vi "Rubix Cube Main.vi"() -> (0 "Rbt cmd":string)   [LabVIEW 2019]
uses:
  left arrow.ctl
  down arrow.ctl
  right arrow.ctl
  up arrow.ctl
  rotate right.ctl
  rotate left.ctl
  TCP send commands.ctl
  UI Mode.ctl
  error module commands.ctl
  Stop Timing Module commands.vi
  main queue data type.ctl
  top level commands.ctl
  Cube Data Ops.ctl
  facet and command.ctl
  Play timing module commands.ctl
  Scene Commands.ctl
  Robot Movement Command Interpreter - to robot.vi
  preform rotate op -numeric.vi
  Robot Movement Command Interpreter - to rubix.vi
panel:
  out "Array":u16[][](array[numeric])=[[1, 5, 2, 4, 3, 5, 4, 2, 3], [0, 5, 4, 1, 2, 0, 5, 2, 2], [1, 2, 1, 1, 0, 0, 4, 1, 4], [3, 4, 0, 4, 1, 1, 2, 4, 3], [5, 3, 0, 2, 5, 3, 5, 0, 5], [1, 5, 2, 3, 4, 0, 0, 3, 3]]
  in  "Sync to Cube":bool
  in  "Rotation Resolution":dbl=10.0
  in  "Go To face":bool
  in  "Solve":bool
  in  "Test":bool
  in  "Difficulty":u16(ring)=5 items=["Easy"=5, "Medium"=20, "Hard"=50, "Challenge"=100]
  in  "Randomize":bool
  in  "Game Play Type":enum16{"Standalone", "UI Master", "UI Salve"}(ring)
  in  "Face":u8=1 min=1 max=6 step=1
  in  "Face ccw":T1
  in  "Face cw":T2
  in  "Right column up":T3
  in  "Middle column up":T3
  in  "Left column up":T3
  in  "Bottom row right":T4
  in  "Middle row right":T4
  in  "Top row right":T4
  in  "Right column down":T5
  in  "Middle column down":T5
  in  "Left column down":T5
  in  "Bottom row left":T6
  in  "Middle row left":T6
  in  "Top row left":T6
  in  "stop":bool
  # "Aux Functions (do not use)"
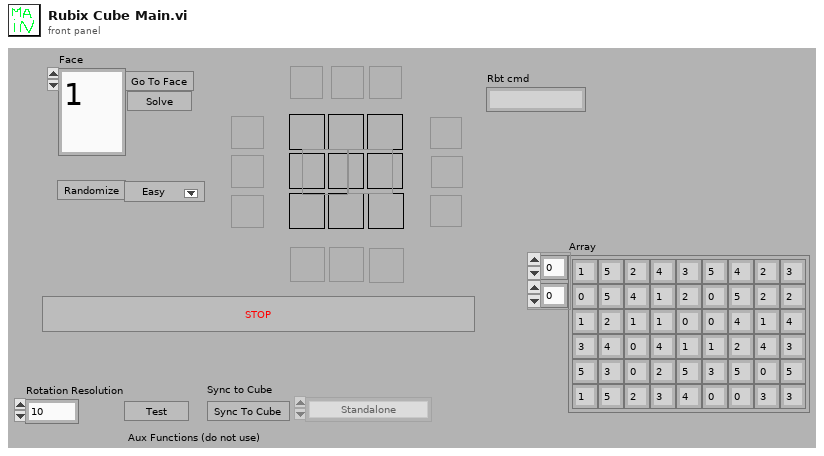
[diagram p1: front panel]
types:
  T1 = typedef "rotate left.ctl" = bool
  T2 = typedef "rotate right.ctl" = bool
  T3 = typedef "up arrow.ctl" = bool
  T4 = typedef "right arrow.ctl" = bool
  T5 = typedef "down arrow.ctl" = bool
  T6 = typedef "left arrow.ctl" = bool
  T7 = typedef "error module commands.ctl" = enum16{"Cleanup References", "Set References", "Report Errors", "Process Errors"}
  T8 = typedef "UI Mode.ctl" = enum16{"Standalone", "UI Master", "UI Salve"}
  T9 = typedef "TCP send commands.ctl" = enum16{"Init TCP", "Close TCP & Stop", "TCP Connected", "Close TCP & Init"}
  T10 = typedef "Main VI references.ctl" = cluster{"Cmd Usr Event":refnum<user-event>, "Event Reg Refnum":refnum<event-registration>, "L1-2 Q":refnum<queue>, "L2-3 Q":refnum<queue>, "Game Play Type":refnum<vi>, "L3-4 Q":refnum<queue>, "Stop Usr Event":refnum<user-event>}
  T11 = typedef "facet and command.ctl" = cluster{"Rotate command":T12, "Facet to act on":u8}
  T12 = typedef "Cube Data Ops.ctl" = enum16{"Initialize", "Set Rubix Ref Array", "Set Rubix Text Array", "Set Current Face", "Get Rubix Text Array", "Generate Rubix Array", "Get Rubix array", "Get Facets to move", "Randomize", "Top row left", "Top row right", "Middle row left", "Middle row right", "Bottom row left", "Bottom row right", "Left column up", "Left column down", "Middle column up", "Middle column down", "Right column up", "Right column down", "Face ccw", "Face cw"}
  T13 = typedef "main queue data type.ctl" = cluster{"Command":T14, "Data":variant}
  T14 = typedef "top level commands.ctl" = enum16{"Idle", "Set Cube Orientation", "Get Cube Orientation", "Go to Face", "Solve", "Test", "Randomize", "Game Play Type", "Stop", "rotate Cube"}
  T15 = typedef "Stop Timing Module commands.vi" = enum16{"Set Name", "Stop loops"}
  T16 = typedef "Play timing module commands.ctl" = enum16{"Clean up", "Initialize", "Run"}
  T17 = typedef "Scene Commands.ctl" = enum16{"Init", "Set Rubix Text Array", "Get Rubix Ref Array", "Generate Rubix Array", "Get Rubix Array", "Show Render Window", "Go To Face", "Rotate", "Update Scene", "Clear Rubix"}
  T18 = typedef "Rubix Array data type.ctl" = cluster{"Object Ref":refnum<vi>, "Name":string}
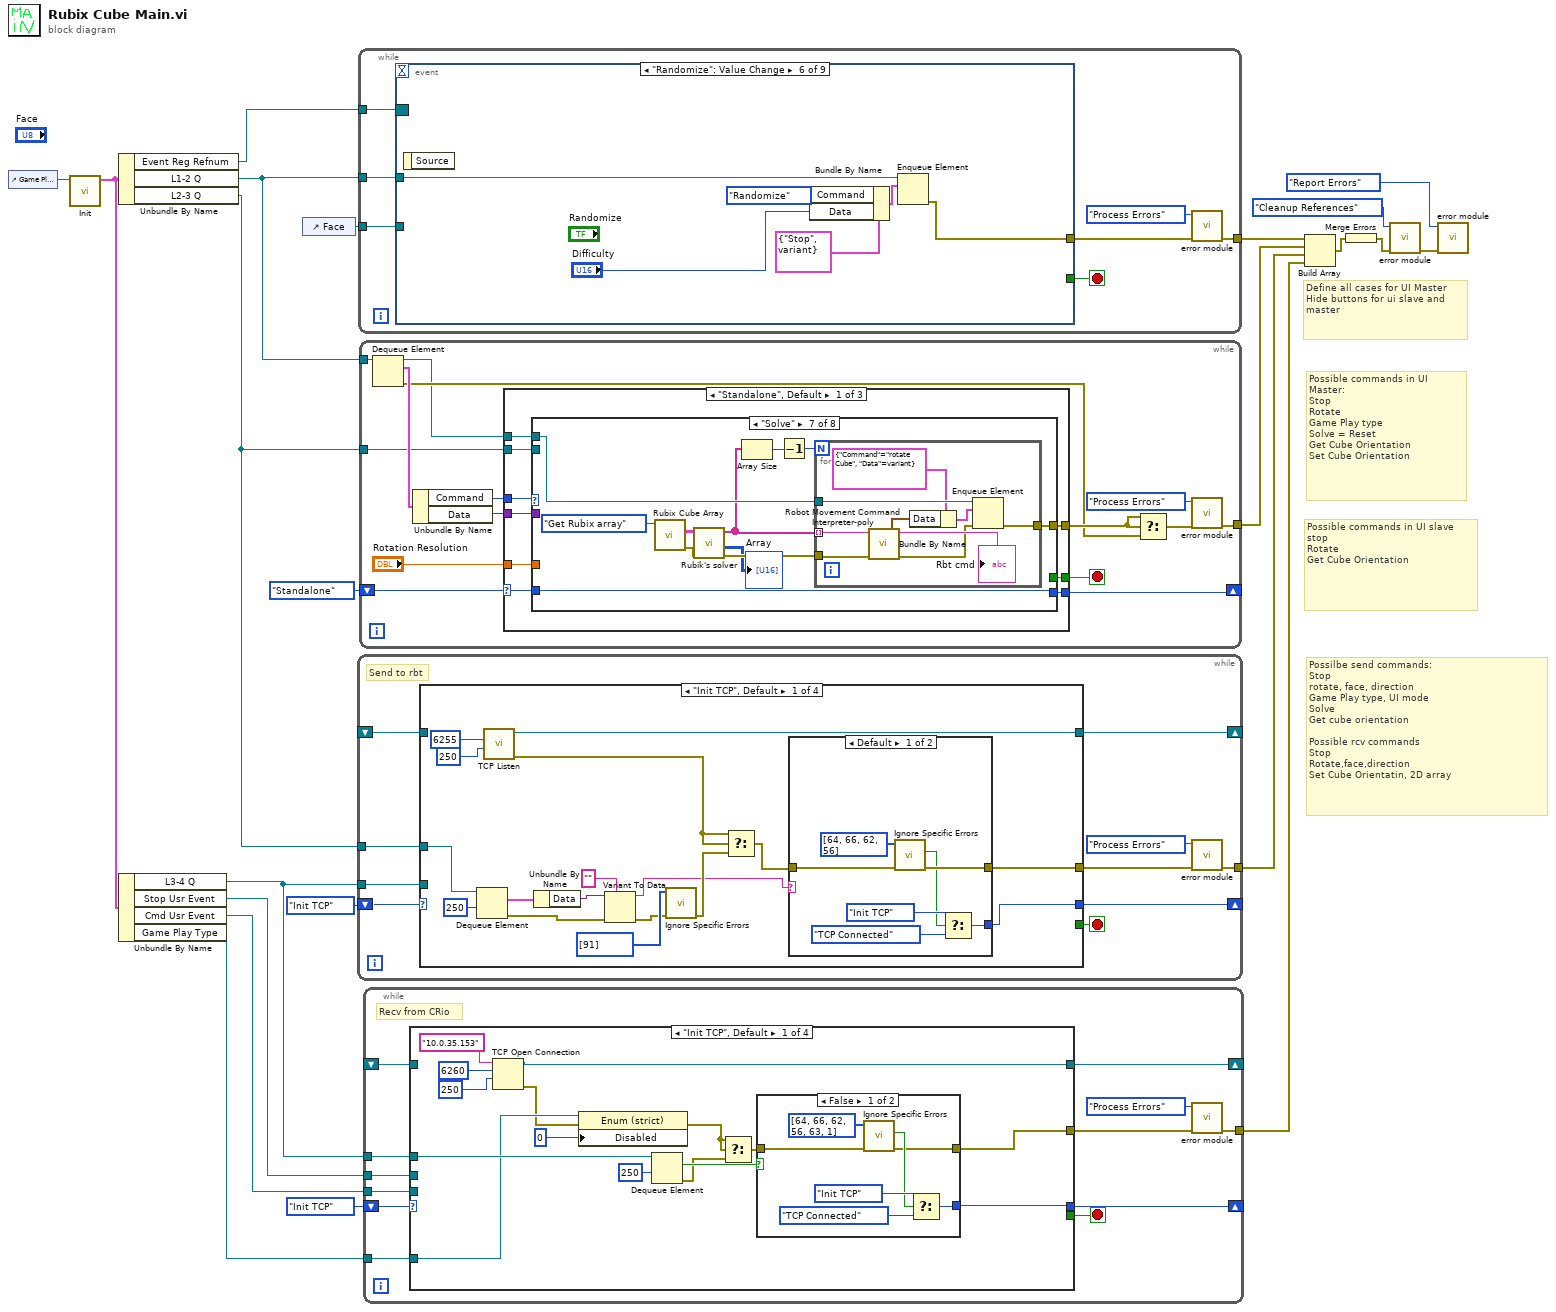
[diagram p0: block diagram]
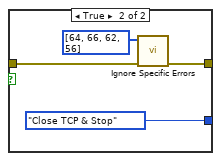
[diagram p2: hidden frame]
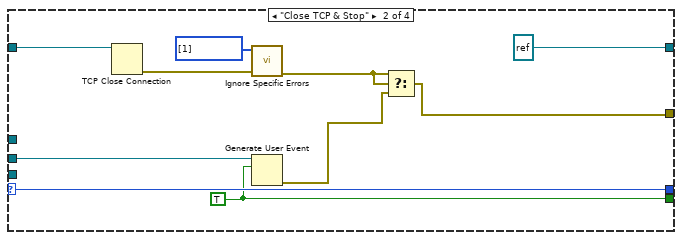
[diagram p3: hidden frame]
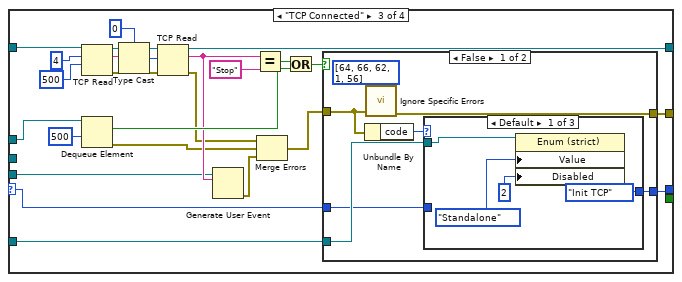
[diagram p4: hidden frame]
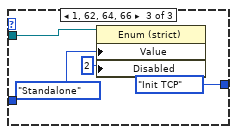
[diagram p6: hidden frame]
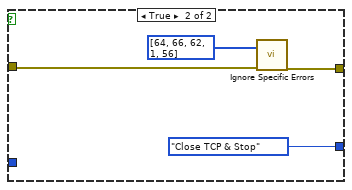
[diagram p7: hidden frame]
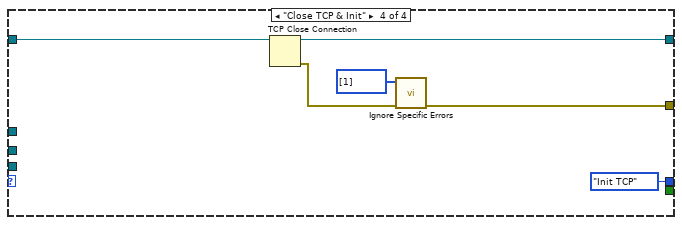
[diagram p8: hidden frame]
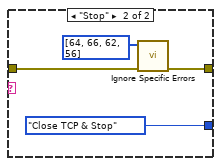
[diagram p9: hidden frame]
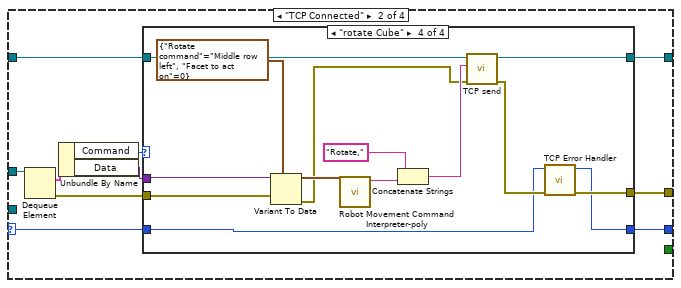
[diagram p10: hidden frame]
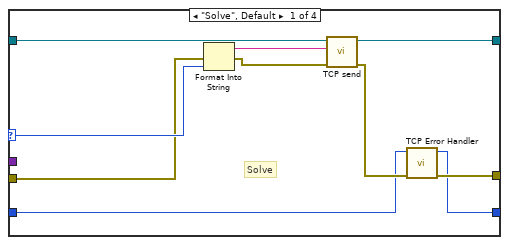
[diagram p11: hidden frame]
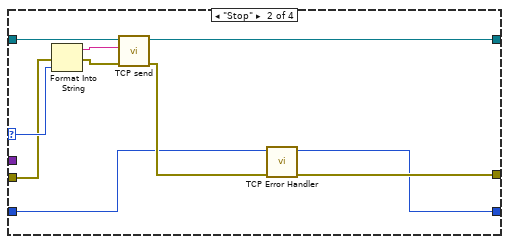
[diagram p12: hidden frame]
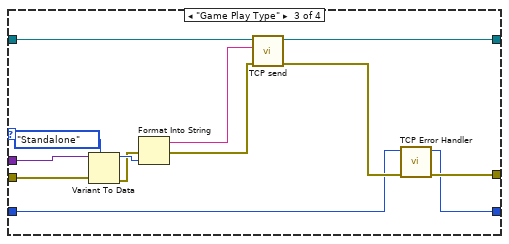
[diagram p13: hidden frame]
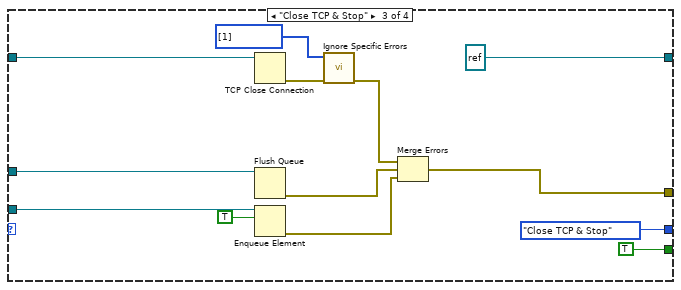
[diagram p14: hidden frame]
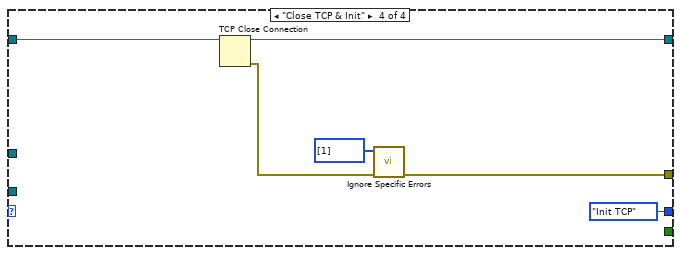
[diagram p15: hidden frame]
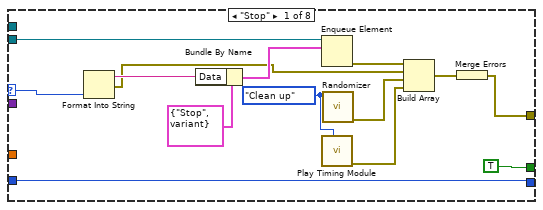
[diagram p16: hidden frame]
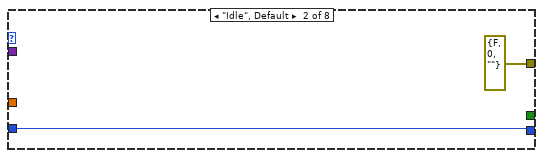
[diagram p17: hidden frame]
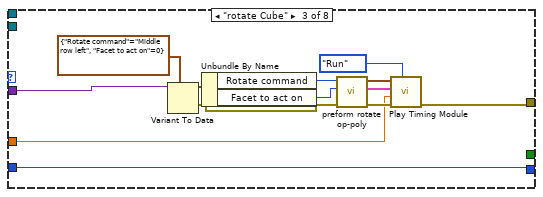
[diagram p18: hidden frame]
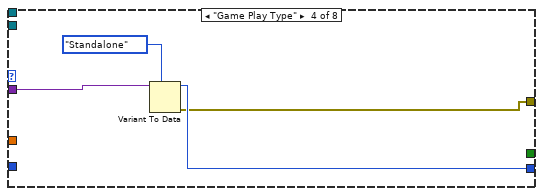
[diagram p19: hidden frame]
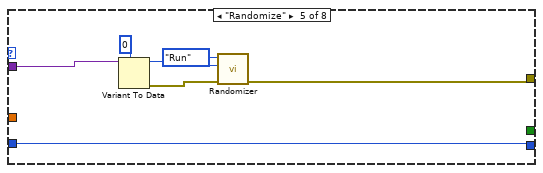
[diagram p20: hidden frame]
diagram:
  # "Possible commands in UI slave\nstop\nRotate\nGet Cube Orientation"
  # "Possible commands in UI Master:\nStop\nRotate\nGame Play type\nSolve = Reset\nGet Cube Orientation\nSet Cube Orientation"
  # "Possilbe send commands:\nStop\nrotate, face, direction\nGame Play type, UI mode\nSolve\nGet cube orientation\n\nPossible rcv commands\nStop\nRotate,face,direction\nSet Cube Orientatin, 2D array"
  # "Define all cases for UI Master\nHide buttons for ui slave and master"
  n1 = control-ref of="Game Play Type"() -> (w18:refnum<vi>)
  n2 = call "Init.vi"("Game Play Type"=w18) -> ("cluster out"=w2:T10)  [unwired: 10 in]
  n3 = Unbundle By Name(w2) -> ("Event Reg Refnum"=w17:refnum<event-registration>, "L1-2 Q"=w16:refnum<queue>, "L2-3 Q"=w15:refnum<queue>)
  n4 = Unbundle By Name(w2) -> ("L3-4 Q"=w14:refnum<queue>, "Stop Usr Event"=w12:refnum<user-event>, "Cmd Usr Event"=w13:refnum<user-event>, "Game Play Type"=w1:refnum<vi>)
  n5 = control-ref of="Face"() -> (w22:refnum<vi>)
  n6 = while {
    shift-right: [w32] -> _
    shift-left: _ -> [w29]
    shift-right: [w31] -> _
    shift-left: TCP_send_commands."Init TCP" ("Enum") -> [w23]
    tunnel: w14 -> [w28]
    tunnel: w15 -> [w27]
    tunnel: [w24] -> w7
    stop <- w30 stop-if-true
    # "Send to rbt"
    n7 = case shown="\"Init TCP\", Default" w23 {
      selector: w23 -> [_ w63 _ _]
      tunnel: [w46 w65 refnum<k5> refnum ("connection ID") w134] -> w32
      tunnel: [w41 w67 TCP_send_commands."Close TCP & Stop" ("Enum") TCP_send_commands."Init TCP" ("Enum")] -> w31
      tunnel: [_ _ TRUE _] -> w30
      tunnel: w29 -> [_ w66 w128 w135]
      tunnel: w28 -> [_ _ w126 _]
      tunnel: w27 -> [w47 w64 w125 _]
      tunnel: [w40 w62 w118 w131] -> w25
      frame "Init TCP", Default {
        n8 = Dequeue Element(queue=w47, timeout in ms (-1)=250) -> (element=w49:T13, error out=w37:errorcluster)  [unwired: 1 in, 2 out]
        n9 = call <vilib>:"TCP Listen.vi"("timeout ms (wait forever: -1)"=250 ("timeout ms (60000)"), "port"=u16 6255 ("remote port")) -> ("error out"=w43:errorcluster, "connection ID"=w46:refnum<k5>)  [unwired: 5 in, 3 out]
        n10 = Unbundle By Name(w49) -> ("Data"=w36:variant)
        n11 = Variant To Data(error in=w37, type="" ("resulting string"), Variant=w36) -> (data=w35:string, error out=w33:errorcluster)
        n12 = call "Ignore Specific Errors.vi"("error in (no error)"=w33, "Array"=i32[] [91]) -> ("error out"=w39:errorcluster)  [unwired: 8 in, 1 out]
        n13 = Select(t=w43, s=w43, f=w39) -> (s? t:f=w42:errorcluster)
        n14 = case shown="Default" w35 {
          tunnel: w42 -> [w52 w58]
          tunnel: [w56 TCP_send_commands."Close TCP & Stop" ("Enum")] -> w41
          tunnel: [w51 w57] -> w40
          frame Default {
            n15 = call "Ignore Specific Errors.vi"("error in (no error)"=w52, "Array"=i32[] [64, 66, 62, 56]) -> ("error out"=w51:errorcluster, "In List?"=w50:bool)  [unwired: 8 in]
            n16 = Select(t=TCP_send_commands."Init TCP" ("Enum"), s=w50, f=TCP_send_commands."TCP Connected" ("Enum")) -> (s? t:f=w56:T9)
          }
          frame "Stop" {
            n17 = call "Ignore Specific Errors.vi"("error in (no error)"=w58, "Array"=i32[] [64, 66, 62, 56]) -> ("error out"=w57:errorcluster)  [unwired: 8 in, 1 out]
          }
        }
      }
      frame "TCP Connected" {
        n18 = Dequeue Element(queue=w64) -> (element=w70:T13, error out=w61:errorcluster)  [unwired: 2 in, 2 out]
        n19 = Unbundle By Name(w70) -> ("Command"=w69:T14, "Data"=w68:variant)
        n20 = case shown="\"rotate Cube\"" w69 {
          selector: w69 -> [w78 w90 _ _]
          tunnel: w68 -> [_ _ w103 w117]
          tunnel: [w72 w82 w93 w105] -> w67
          tunnel: w66 -> [w80 w89 w101 w116]
          tunnel: [w79 w88 w100 w115] -> w65
          tunnel: w63 -> [w73 w83 w92 w106]
          tunnel: [w74 w85 w94 w107] -> w62
          tunnel: w61 -> [w71 w81 w91 w104]
          frame "Solve", Default {
            # "Solve"
            n21 = Format Into String(error in=w71, w78) -> (resulting string=w77:string, error out=w76:errorcluster)  [unwired: 2 in]
            n22 = call "TCP send.vi"("error in (no error)"=w76, "string"=w77, "connection ID in"=w80) -> ("error out"=w75:errorcluster, "connection ID out"=w79:refnum<k5>)  [unwired: 7 in]
            n23 = call "TCP Error Handler.vi"("Error In"=w75, "TCP State In"=w73) -> ("error out"=w74:errorcluster, "TCP State Out"=w72:T9)  [unwired: 8 in]
          }
          frame "Stop" {
            n24 = Format Into String(error in=w81, w90) -> (resulting string=w87:string, error out=w86:errorcluster)  [unwired: 2 in]
            n25 = call "TCP send.vi"("error in (no error)"=w86, "string"=w87, "connection ID in"=w89) -> ("error out"=w84:errorcluster, "connection ID out"=w88:refnum<k5>)  [unwired: 7 in]
            n26 = call "TCP Error Handler.vi"("Error In"=w84, "TCP State In"=w83) -> ("error out"=w85:errorcluster, "TCP State Out"=w82:T9)  [unwired: 8 in]
          }
          frame "Game Play Type" {
            n27 = Variant To Data(error in=w91, type=UI_Mode."Standalone" ("Game Play Type 2"), Variant=w103) -> (data=w99:T8, error out=w97:errorcluster)
            n28 = Format Into String(error in=w97, w99) -> (resulting string=w98:string, error out=w96:errorcluster)  [unwired: 2 in]
            n29 = call "TCP send.vi"("error in (no error)"=w96, "string"=w98, "connection ID in"=w101) -> ("error out"=w95:errorcluster, "connection ID out"=w100:refnum<k5>)  [unwired: 7 in]
            n30 = call "TCP Error Handler.vi"("Error In"=w95, "TCP State In"=w92) -> ("error out"=w94:errorcluster, "TCP State Out"=w93:T9)  [unwired: 8 in]
          }
          frame "rotate Cube" {
            n31 = Variant To Data(error in=w104, type=T11 {"Rotate command"=enum."Middle row left", "Facet to act on"=0} ("Cluster"), Variant=w117) -> (data=w113:T11, error out=w109:errorcluster)
            n32 = call-poly "Robot Movement Command Interpreter-poly.vi"("Rubix Cmd"=w113) -> ("Rbt Cmd"=w112:string)  [unwired: 10 in]
            n33 = Concatenate Strings("Rotate," ("string"), w112) -> (w110:string)
            n34 = call "TCP send.vi"("error in (no error)"=w109, "string"=w110, "connection ID in"=w116) -> ("error out"=w108:errorcluster, "connection ID out"=w115:refnum<k5>)  [unwired: 7 in]
            n35 = call "TCP Error Handler.vi"("Error In"=w108, "TCP State In"=w106) -> ("error out"=w107:errorcluster, "TCP State Out"=w105:T9)  [unwired: 8 in]
          }
        }
      }
      frame "Close TCP & Stop" {
        n36 = TCP Close Connection(connection ID=w128) -> (error out=w122:errorcluster)  [unwired: 2 in, 1 out]
        n37 = Flush Queue(queue=w125) -> (error out=w120:errorcluster)  [unwired: 1 in, 2 out]
        n38 = Enqueue Element(queue=w126, element=TRUE) -> (error out=w119:errorcluster)  [unwired: 2 in, 2 out]
        n39 = call "Ignore Specific Errors.vi"("error in (no error)"=w122, "Array"=i32[] [1]) -> ("error out"=w121:errorcluster)  [unwired: 8 in, 1 out]
        n40 = Merge Errors(w121, w120, w119) -> (w118:errorcluster)
      }
      frame "Close TCP & Init" {
        n41 = TCP Close Connection(connection ID=w135) -> (connection ID out=w134:refnum<k5>, error out=w132:errorcluster)  [unwired: 2 in]
        n42 = call "Ignore Specific Errors.vi"("error in (no error)"=w132, "Array"=i32[] [1]) -> ("error out"=w131:errorcluster)  [unwired: 8 in, 1 out]
      }
    }
    n43 = call "error module.vi"("error in (no error)"=w25, "Enum"=error_module_commands."Process Errors") -> ("error out"=w24:errorcluster)  [unwired: 9 in]
  }
  n44 = while {
    tunnel: w16 -> [w143]
    tunnel: w22 -> [w141]
    tunnel: w17 -> [w140]
    tunnel: [w138] -> w9
    stop <- w142 stop-if-true
    n45 = event shown="[5] \"Randomize\": Value Change" {
      selector: w140 -> [_ _ _ _ _ _ _ _ _]
      dyn-events: _ -> [_ _ _ _ _ _ _ _ _]
      timeout: _ -> [_ _ _ _ _ _ _ _ _]
      tunnel: w143 -> [w150 w156 w160 w162 w166 w169 w175 w186 w193]
      tunnel: [TRUE ("stop") _ _ _ _ _ _ _ _] -> w142
      tunnel: [w146 w153 w159 w161 w164 w168 w173 w185 w189] -> w139
      tunnel: w141 -> [_ w155 _ _ _ _ _ w184 _]
      event User Event; "stop": Value Change {
        n46 = event-data() -> ()  [unwired: 1 in, 1 out]
        n47 = call "Stop Timing Module.vi"("command"=Stop_Timing_Module_commands.vi."Stop loops") -> ("error out"=w147:errorcluster)  [unwired: 10 in]
        n48 = Enqueue Element At Opposite End(queue=w150, element=T13 {"Command"=enum."Stop", "Data"=variant} ("Cluster")) -> (error out=w148:errorcluster)  [unwired: 2 in, 2 out]
        n49 = Select(t=w148, s=w148, f=w147) -> (s? t:f=w146:errorcluster)
      }
      event "Go To face": Value Change {
        n50 = event-data() -> ()  [unwired: 1 in, 1 out]
        n51 = property class="DigNum (strict)"(reference=w155) -> (error out=w152:errorcluster, "Value"=w154:u8)  [unwired: 1 in, 1 out]
        n52 = Bundle By Name(cluster=T13 {"Command"=enum."Go to Face", "Data"=variant} ("Cluster"), "Data"=w154) -> (w157:T13)
        n53 = Enqueue Element(queue=w156, element=w157, error in (no error)=w152) -> (error out=w153:errorcluster)  [unwired: 1 in, 2 out]
      }
      event "Solve": Value Change {
        n54 = event-data() -> ()  [unwired: 1 in, 1 out]
        n55 = Enqueue Element(queue=w160, element=T13 {"Command"=enum."Solve", "Data"=variant} ("Cluster")) -> (error out=w159:errorcluster)  [unwired: 2 in, 2 out]
      }
      event User Event {
        # "interpret string based on command"
        n56 = event-data() -> ("Command"=w163:string)  [unwired: 1 in]
        n57 = call "Command Interpreter.vi"("Command"=w163, "L1-2 Q"=w162) -> ("error out"=w161:errorcluster)  [unwired: 8 in, 1 out]
      }
      event "Sync to Cube": Value Change {
        n58 = event-data() -> ()  [unwired: 1 in, 1 out]
        n59 = Enqueue Element(queue=w166, element=T13 {"Command"=enum."Get Cube Orientation", "Data"=variant} ("Cluster")) -> (error out=w164:errorcluster)  [unwired: 2 in, 2 out]
      }
      event "Randomize": Value Change {
        n60 = event-data() -> ()  [unwired: 1 in, 1 out]
        n61 = Bundle By Name(cluster=T13 {"Command"=enum."Stop", "Data"=variant} ("Cluster"), "Command"=top_level_commands."Randomize" ("Enum"), "Data"="Difficulty") -> (w172:T13)
        n62 = Enqueue Element(queue=w169, element=w172) -> (error out=w168:errorcluster)  [unwired: 2 in, 2 out]
      }
      event "Test": Value Change {
        n63 = event-data() -> ()  [unwired: 1 in, 1 out]
        n64 = Enqueue Element(queue=w175, element=T13 {"Command"=enum."Test", "Data"=variant} ("Cluster")) -> (error out=w173:errorcluster)  [unwired: 2 in, 2 out]
      }
      event Value Change {
        n65 = event-data() -> ("CtlRef"=w180:refnum<vi>)  [unwired: 1 in]
        n66 = property class="DigNum (strict)"(reference=w184) -> ("Value"=w182:u8)  [unwired: 1 in, 2 out]
        n67 = property class="Bool"(reference=w180) -> ("Label.Text"=w178:string)  [unwired: 1 in, 2 out]
        n68 = Scan From String(input string=w178, default 1=Cube_Data_Ops."Right column up" ("Rotate command")) -> (error out=w176:errorcluster, output 1=w177:T12)  [unwired: 3 in, 2 out]
        n69 = Bundle By Name(cluster=T11 {"Rotate command"=enum."Middle row left", "Facet to act on"=0} ("Cluster"), "Rotate command"=w177, "Facet to act on"=w182) -> (w181:T11)
        n70 = Bundle By Name(cluster=T13 {"Command"=enum."rotate Cube", "Data"=variant} ("Cluster"), "Data"=w181) -> (w188:T13)
        n71 = Enqueue Element(queue=w186, element=w188, error in (no error)=w176) -> (error out=w185:errorcluster)  [unwired: 1 in, 2 out]
      }
      event "Game Play Type": Value Change {
        n72 = event-data() -> ()  [unwired: 1 in, 1 out]
        n73 = Bundle By Name(cluster=T13 {"Command"=enum."Game Play Type", "Data"=variant} ("Cluster"), "Data"="Game Play Type") -> (w190:T13)
        n74 = Enqueue Element(queue=w193, element=w190) -> (error out=w189:errorcluster)  [unwired: 2 in, 2 out]
      }
    }
    n75 = call "error module.vi"("error in (no error)"=w139, "Enum"=error_module_commands."Process Errors") -> ("error out"=w138:errorcluster)  [unwired: 9 in]
  }
  n76 = while {
    tunnel: w16 -> [w208]
    shift-right: [w203] -> _
    shift-left: UI_Mode."Standalone" ("Game Play Type 2") -> [w204]
    tunnel: w15 -> [w202]
    tunnel: [w201] -> w8
    stop <- w205 stop-if-true
    n77 = Dequeue Element(queue=w208) -> (queue out=w196:refnum<queue>, element=w207:T13, error out=w198:errorcluster)  [unwired: 2 in, 1 out]
    n78 = Unbundle By Name(w207) -> ("Command"=w195:T14, "Data"=w206:variant)
    n79 = case shown="\"Standalone\", Default" w204 {
      selector: w204 -> [w214 w313 w384]
      tunnel: w195 -> [w217 w310 w386]
      tunnel: w206 -> [w216 w312 w385]
      tunnel: [w215 w315 w383] -> w205
      tunnel: [w213 w314 w382] -> w203
      tunnel: w202 -> [w212 w311 w387]
      tunnel: [w211 w309 w381] -> w199
      tunnel: w196 -> [w210 _ _]
      tunnel: "Rotation Resolution" -> [w209 w308 w380]
      frame "Standalone", Default {
        n80 = case shown="\"Solve\"" w217 {
          selector: w217 -> [w227 _ _ _ _ _ _ _]
          tunnel: [TRUE _ _ _ _ _ _ _] -> w215
          tunnel: w216 -> [_ _ w246 w250 w257 _ _ w307]
          tunnel: w214 -> [w229 w233 w238 _ w253 w260 w290 w301]
          tunnel: [w229 w233 w238 w249 w253 w260 w290 w301] -> w213
          tunnel: w212 -> [w228 _ _ _ _ _ _ _]
          tunnel: [w223 errorcluster {"status"=FALSE, "code"=0, "source"=""} ("error out") w237 w247 w251 w259 w288 w299] -> w211
          tunnel: w210 -> [_ _ _ _ _ _ w286 _]
          tunnel: w209 -> [_ _ w234 _ _ w258 _ _]
          frame "Stop" {
            w230 = Play_timing_module_commands."Clean up" ("Commands")
            n81 = Format Into String(w227) -> (resulting string=w225:string, error out=w220:errorcluster)  [unwired: 3 in]
            n82 = Bundle By Name(cluster=T13 {"Command"=enum."Stop", "Data"=variant} ("Cluster"), "Data"=w225) -> (w224:T13)
            n83 = Enqueue Element(queue=w228, element=w224) -> (error out=w222:errorcluster)  [unwired: 2 in, 2 out]
            n84 = call "Play Timing Module.vi"("Commands"=w230) -> ("error out"=w218:errorcluster)  [unwired: 10 in]
            n85 = call "Randomizer.vi"("Commands"=w230) -> ("error out"=w219:errorcluster)  [unwired: 9 in, 1 out]
            n86 = Build Array(w222, w220, w219, w218) -> (w221:errorcluster[])
            n87 = Merge Errors(w221) -> (w223:errorcluster)
          }
          frame "Idle", Default {
          }
          frame "rotate Cube" {
            n88 = Variant To Data(type=T11 {"Rotate command"=enum."Middle row left", "Facet to act on"=0} ("Cluster"), Variant=w246) -> (data=w241:T11, error out=w235:errorcluster)  [unwired: 1 in]
            n89 = Unbundle By Name(w241) -> ("Rotate command"=w240:T12, "Facet to act on"=w239:u8)
            n90 = call-poly "preform rotate op-poly.vi"("error in (no error)"=w235, "Face to act on"=w239, "Rotate command"=w240) -> ("error out(no error)"=w236:errorcluster, "Facets To move"=w243:T18[], "Axis"=w244:cluster{"X":sgl, "Y":sgl, "Z":sgl})  [unwired: 6 in]
            n91 = call "Play Timing Module.vi"("Commands"=Play_timing_module_commands."Run", "error in"=w236, "Rotation Resolution"=w234, "Facets To move"=w243, "Axis"=w244) -> ("error out"=w237:errorcluster)  [unwired: 6 in]
          }
          frame "Game Play Type" {
            n92 = Variant To Data(type=UI_Mode."Standalone" ("Game Play Type 2"), Variant=w250) -> (data=w249:T8, error out=w247:errorcluster)  [unwired: 1 in]
          }
          frame "Randomize" {
            n93 = Variant To Data(type=0, Variant=w257) -> (data=w255:i32, error out=w252:errorcluster)  [unwired: 1 in]
            n94 = call "Randomizer.vi"("error in"=w252, "Difficulty"=w255, "Commands"=Play_timing_module_commands."Run") -> ("error out"=w251:errorcluster)  [unwired: 7 in, 1 out]
          }
          frame "Test" {
            n95 = for {
              N: 6 -> [_]
              tunnel: [w263] -> w259
              tunnel: w258 -> [w262]
              i -> [w265]
              n96 = Increment(x=w265) -> (x+1=w264:i32)
              n97 = for {
                N: 14 -> [_]
                tunnel: w264 -> [w269]
                tunnel: [w268] -> w263
                tunnel: w262 -> [w267]
                i -> [w271]
                n98 = Add(x=w271, y=9) -> (x+y=w272:i32)
                n99 = To Word Integer(number=w272) -> (16bit integer=w273:i16)
                n100 = Type Cast(type=Cube_Data_Ops."Top row left" ("Rotate command"), x=w273) -> (*(type *) &x=w270:T12)
                n101 = call-poly "preform rotate op-poly.vi"("Face to act on"=w269, "Rotate command"=w270) -> ("error out(no error)"=w279:errorcluster, "Facets To move"=w278:T18[], "Axis"=w277:cluster{"X":sgl, "Y":sgl, "Z":sgl})  [unwired: 7 in]
                n102 = call "Play Timing Module.vi"("Commands"=Play_timing_module_commands."Run", "error in"=w279, "Rotation Resolution"=w267, "Facets To move"=w278, "Axis"=w277) -> ("error out"=w268:errorcluster)  [unwired: 6 in]
              }
            }
          }
          frame "Solve" {
            n103 = call "Rubix Cube Array.vi"("Command"=Cube_Data_Ops."Get Rubix array") -> ("error out(no error)"=w281:errorcluster, "Rubix Array"=w287:T18[][])  [unwired: 6 in, 3 out]
            n104 = call "Rubik's solver.vi"("error in (no error)"=w281, "Rubix Array"=w287) -> ("error out"=w282:errorcluster, "Array"=→"Array":u16[][], "Commands to Execute"=w285:string[])  [unwired: 6 in, 1 out]
            n105 = Array Size(array=w285) -> (size(s)=w284:i32)
            n106 = Decrement(x=w284) -> (x-1=w283:i32)
            n107 = for {
              N: w283 -> [_]
              tunnel: w286 -> [w298]
              tunnel: w285 -> [w294] mode=indexing
              tunnel: [w295] -> w288
              tunnel: w282 -> [w291]
              n108 = call-poly "Robot Movement Command Interpreter-poly.vi"("error in (no error)"=w291, "Rbt Cmd"=w294) -> ("error out"=w292:errorcluster, "Rubix Cmd"=w293:T11)  [unwired: 7 in, 1 out]
              n109 = Bundle By Name(cluster=T13 {"Command"=enum."rotate Cube", "Data"=variant} ("element"), "Data"=w293) -> (w296:T13)
              n110 = Enqueue Element(queue=w298, element=w296, error in (no error)=w292) -> (error out=w295:errorcluster)  [unwired: 1 in, 2 out]
              "Rbt cmd" <- w294
            }
          }
          frame "Go to Face" {
            n111 = Variant To Data(type=u8 0 ("Value"), Variant=w307) -> (data=w304:u8, error out=w300:errorcluster)  [unwired: 1 in]
            n112 = call "Scene func global.vi"("Face of interest"=w304, "error in (no error)"=w300, "Commands"=Scene_Commands."Go To Face") -> ("error out"=w303:errorcluster)  [unwired: 7 in, 1 out]
            n113 = call "Scene func global.vi"("error in (no error)"=w303, "Commands"=Scene_Commands."Update Scene") -> ("error out"=w299:errorcluster)  [unwired: 8 in, 1 out]
          }
        }
      }
      frame "UI Master" {
        n114 = case shown="\"Stop\"" w310 {
          selector: w310 -> [w322 _ _ _ w364 _ _]
          tunnel: [TRUE _ _ _ _ _ _] -> w315
          tunnel: w312 -> [_ w347 w356 _ _ _ w376]
          tunnel: w313 -> [w327 w342 _ w360 w369 w371 w377]
          tunnel: [w327 w342 w351 w360 w369 w371 w377] -> w314
          tunnel: w311 -> [w326 w341 w354 w359 w365 _ _]
          tunnel: [w316 w332 w348 w357 w362 errorcluster {"status"=FALSE, "code"=0, "source"=""} ("error IO") w373] -> w309
          tunnel: w308 -> [_ w330 _ _ _ _ _]
          frame "Stop" {
            w328 = Play_timing_module_commands."Clean up" ("Commands")
            n115 = Format Into String(w322) -> (resulting string=w324:string, error out=w320:errorcluster)  [unwired: 3 in]
            n116 = Bundle By Name(cluster=T13 {"Command"=enum."Stop", "Data"=variant} ("Cluster"), "Data"=w324) -> (w323:T13)
            n117 = Enqueue Element(queue=w326, element=w323) -> (error out=w321:errorcluster)  [unwired: 2 in, 2 out]
            n118 = call "Randomizer.vi"("Commands"=w328) -> ("error out"=w319:errorcluster)  [unwired: 9 in, 1 out]
            n119 = call "Play Timing Module.vi"("Commands"=w328) -> ("error out"=w318:errorcluster)  [unwired: 10 in]
            n120 = Build Array(w321, w320, w319, w318) -> (w317:errorcluster[])
            n121 = Merge Errors(w317) -> (w316:errorcluster)
          }
          frame "rotate Cube" {
            n122 = Variant To Data(type=T11 {"Rotate command"=enum."Middle row left", "Facet to act on"=0} ("Cluster"), Variant=w347) -> (data=w336:T11, error out=w334:errorcluster)  [unwired: 1 in]
            n123 = Unbundle By Name(w336) -> ("Rotate command"=w337:T12, "Facet to act on"=w338:u8)
            n124 = Bundle By Name(cluster=T13 {"Command"=enum."rotate Cube", "Data"=variant} ("element"), "Data"=w336) -> (w339:T13)
            n125 = call-poly "preform rotate op-poly.vi"("error in (no error)"=w334, "Face to act on"=w338, "Rotate command"=w337) -> ("error out(no error)"=w335:errorcluster, "Facets To move"=w344:T18[], "Axis"=w345:cluster{"X":sgl, "Y":sgl, "Z":sgl})  [unwired: 6 in]
            n126 = Enqueue Element(queue=w341, element=w339) -> (error out=w333:errorcluster)  [unwired: 2 in, 2 out]
            n127 = call "Play Timing Module.vi"("Commands"=Play_timing_module_commands."Run", "error in"=w335, "Rotation Resolution"=w330, "Facets To move"=w344, "Axis"=w345) -> ("error out"=w331:errorcluster)  [unwired: 6 in]
            n128 = Select(t=w333, s=w333, f=w331) -> (s? t:f=w332:errorcluster)
          }
          frame "Game Play Type" {
            n129 = Variant To Data(type=UI_Mode."Standalone" ("Game Play Type 2"), Variant=w356) -> (data=w351:T8, error out=w349:errorcluster)  [unwired: 1 in]
            n130 = Bundle By Name(cluster=T13 {"Command"=enum."Game Play Type", "Data"=variant} ("element"), "Data"=w351) -> (w352:T13)
            n131 = Enqueue Element(queue=w354, element=w352) -> (error out=w350:errorcluster)  [unwired: 2 in, 2 out]
            n132 = Select(t=w350, s=w350, f=w349) -> (s? t:f=w348:errorcluster)
          }
          frame "Solve" {
            # "fix = input whatever comes from crio"
            n133 = Enqueue Element(queue=w359, element=T13 {"Command"=enum."Solve", "Data"=variant}) -> (error out=w357:errorcluster)  [unwired: 2 in, 2 out]
          }
          frame "Get Cube Orientation" {
            n134 = Format Into String(w364) -> (resulting string=w367:string, error out=w363:errorcluster)  [unwired: 3 in]
            n135 = Bundle By Name(cluster=T13 {"Command"=enum."Get Cube Orientation", "Data"=variant} ("Cluster"), "Data"=w367) -> (w366:T13)
            n136 = Enqueue Element(queue=w365, element=w366) -> (error out=w361:errorcluster)  [unwired: 2 in, 2 out]
            n137 = Select(t=w361, s=w361, f=w363) -> (s? t:f=w362:errorcluster)
          }
          frame "Idle", Default {
          }
          frame "Set Cube Orientation" {
            n138 = Variant To Data(type=string[][] [] ("Rubix array out"), Variant=w376) -> (data=w374:string[][], error out=w372:errorcluster)  [unwired: 1 in]
            n139 = call "Create New Rubix Cube.vi"("error out"=w372, "Rubix Array pattern"=w374) -> ("error out(no error)"=w379:errorcluster)  [unwired: 9 in]
            n140 = call "Scene func global.vi"("error in (no error)"=w379, "Commands"=Scene_Commands."Update Scene") -> ("error out"=w373:errorcluster)  [unwired: 8 in, 1 out]
          }
        }
      }
      frame "UI Salve" {
        n141 = case shown="\"Set Cube Orientation\"" w386 {
          selector: w386 -> [w394 _ _ _ _]
          tunnel: [TRUE _ _ _ _] -> w383
          tunnel: w385 -> [_ _ w406 w424 w433]
          tunnel: w384 -> [w399 w403 w411 w418 _]
          tunnel: [w399 w403 w411 w418 w428] -> w382
          tunnel: w387 -> [w395 _ _ _ w431]
          tunnel: [w388 errorcluster {"status"=FALSE, "code"=0, "source"=""} ("error out") w405 w413 w427] -> w381
          tunnel: w380 -> [_ _ _ w412 _]
          frame "Stop" {
            w400 = Play_timing_module_commands."Clean up" ("Commands")
            n142 = Format Into String(w394) -> (resulting string=w397:string, error out=w392:errorcluster)  [unwired: 3 in]
            n143 = Bundle By Name(cluster=T13 {"Command"=enum."Stop", "Data"=variant} ("Cluster"), "Data"=w397) -> (w396:T13)
            n144 = Enqueue Element(queue=w395, element=w396) -> (error out=w393:errorcluster)  [unwired: 2 in, 2 out]
            n145 = call "Randomizer.vi"("Commands"=w400) -> ("error out"=w391:errorcluster)  [unwired: 9 in, 1 out]
            n146 = call "Play Timing Module.vi"("Commands"=w400) -> ("error out"=w390:errorcluster)  [unwired: 10 in]
            n147 = Build Array(w393, w392, w391, w390) -> (w389:errorcluster[])
            n148 = Merge Errors(w389) -> (w388:errorcluster)
          }
          frame "Idle", Default {
          }
          frame "Set Cube Orientation" {
            n149 = Variant To Data(type=string[][] [] ("Rubix array out"), Variant=w406) -> (data=w407:string[][], error out=w404:errorcluster)  [unwired: 1 in]
            n150 = call "Create New Rubix Cube.vi"("error out"=w404, "Rubix Array pattern"=w407) -> ("error out(no error)"=w410:errorcluster)  [unwired: 9 in]
            n151 = call "Scene func global.vi"("error in (no error)"=w410, "Commands"=Scene_Commands."Update Scene") -> ("error out"=w405:errorcluster)  [unwired: 8 in, 1 out]
          }
          frame "rotate Cube" {
            n152 = Variant To Data(type=T11 {"Rotate command"=enum."Middle row left", "Facet to act on"=0} ("Cluster"), Variant=w424) -> (data=w419:T11, error out=w415:errorcluster)  [unwired: 1 in]
            n153 = Unbundle By Name(w419) -> ("Rotate command"=w416:T12, "Facet to act on"=w417:u8)
            n154 = call-poly "preform rotate op-poly.vi"("error in (no error)"=w415, "Face to act on"=w417, "Rotate command"=w416) -> ("error out(no error)"=w414:errorcluster, "Facets To move"=w421:T18[], "Axis"=w422:cluster{"X":sgl, "Y":sgl, "Z":sgl})  [unwired: 6 in]
            n155 = call "Play Timing Module.vi"("Commands"=Play_timing_module_commands."Run", "error in"=w414, "Rotation Resolution"=w412, "Facets To move"=w421, "Axis"=w422) -> ("error out"=w413:errorcluster)  [unwired: 6 in]
          }
          frame "Game Play Type" {
            n156 = Variant To Data(type=UI_Mode."Standalone" ("Game Play Type 2"), Variant=w433) -> (data=w428:T8, error out=w425:errorcluster)  [unwired: 1 in]
            n157 = Bundle By Name(cluster=T13 {"Command"=enum."Game Play Type", "Data"=variant} ("element"), "Data"=w428) -> (w429:T13)
            n158 = Enqueue Element(queue=w431, element=w429) -> (error out=w426:errorcluster)  [unwired: 2 in, 2 out]
            n159 = Select(t=w426, s=w426, f=w425) -> (s? t:f=w427:errorcluster)
          }
        }
      }
    }
    n160 = Select(t=w199, s=w199, f=w198) -> (s? t:f=w197:errorcluster)
    n161 = call "error module.vi"("error in (no error)"=w197, "Enum"=error_module_commands."Process Errors") -> ("error out"=w201:errorcluster)  [unwired: 9 in]
  }
  n162 = while {
    shift-right: [w444] -> _
    shift-left: TCP_send_commands."Init TCP" ("Enum") -> [w435]
    shift-right: [w443] -> _
    shift-left: _ -> [w442]
    tunnel: w14 -> [w441]
    tunnel: w12 -> [w440]
    tunnel: w13 -> [w439]
    tunnel: w1 -> [w438]
    tunnel: [w436] -> w6
    stop <- w445 stop-if-true
    # "Recv from CRio"
    n163 = case shown="\"Init TCP\", Default" w435 {
      selector: w435 -> [_ w481 w482 _]
      tunnel: [_ w475 _ _] -> w445
      tunnel: [w460 w481 w489 TCP_send_commands."Init TCP" ("Enum")] -> w444
      tunnel: [w450 refnum<k5> refnum ("connection ID") w497 w527] -> w443
      tunnel: w442 -> [_ w480 w506 w531]
      tunnel: w441 -> [w459 _ w503 _]
      tunnel: w440 -> [_ w478 _ _]
      tunnel: w439 -> [_ _ w491 _]
      tunnel: w438 -> [w456 _ w483 _]
      tunnel: [w455 w472 w488 w529] -> w434
      frame "Init TCP", Default {
        n164 = TCP Open Connection(address="10.0.35.153", remote port or service name=u16 6260 ("remote port"), timeout ms (60000)=250) -> (connection ID=w450:refnum<k5>, error out=w454:errorcluster)  [unwired: 2 in]
        n165 = property class="Enum (strict)"(reference=w456, error in=w454, "Disabled"=u8 0) -> (error out=w447:errorcluster)  [unwired: 1 out]
        n166 = Dequeue Element(queue=w459, timeout in ms (-1)=250) -> (element=w458:bool, error out=w448:errorcluster)  [unwired: 1 in, 2 out]
        n167 = Select(t=w447, s=w447, f=w448) -> (s? t:f=w446:errorcluster)
        n168 = case shown="False" w458 {
          tunnel: w446 -> [w462 w469]
          tunnel: [w467 TCP_send_commands."Close TCP & Stop" ("Enum")] -> w460
          tunnel: [w461 w468] -> w455
          frame False {
            n169 = call "Ignore Specific Errors.vi"("error in (no error)"=w462, "Array"=i32[] [64, 66, 62, 56, 63, 1]) -> ("error out"=w461:errorcluster, "In List?"=w463:bool)  [unwired: 8 in]
            n170 = Select(t=TCP_send_commands."Init TCP" ("Enum"), s=w463, f=TCP_send_commands."TCP Connected" ("Enum")) -> (s? t:f=w467:T9)
          }
          frame True {
            n171 = call "Ignore Specific Errors.vi"("error in (no error)"=w469, "Array"=i32[] [64, 66, 62, 56]) -> ("error out"=w468:errorcluster)  [unwired: 8 in, 1 out]
          }
        }
      }
      frame "Close TCP & Stop" {
        w475 = TRUE
        n172 = TCP Close Connection(connection ID=w480) -> (error out=w476:errorcluster)  [unwired: 2 in, 1 out]
        n173 = call "Ignore Specific Errors.vi"("error in (no error)"=w476, "Array"=i32[] [1]) -> ("error out"=w474:errorcluster)  [unwired: 8 in, 1 out]
        n174 = Generate User Event(user event=w478, event data cluster=w475) -> (error out=w473:errorcluster)  [unwired: 2 in, 1 out]
        n175 = Select(t=w474, s=w474, f=w473) -> (s? t:f=w472:errorcluster)
      }
      frame "TCP Connected" {
        n176 = TCP Read(connection ID=w506, bytes to read=4, 9:500 ("timeout ms (25000)")) -> (connection ID out=w498:refnum<k5>, data out=w496:string, error out=w493:errorcluster)  [unwired: 2 in]
        n177 = Dequeue Element(queue=w503, timeout in ms (-1)=500) -> (element=w499:bool, error out=w484:errorcluster)  [unwired: 1 in, 2 out]
        n178 = Type Cast(type=0 ("bytes to read"), x=w496) -> (*(type *) &x=w494:i32)
        n179 = TCP Read(connection ID=w498, bytes to read=w494, error in (no error)=w493) -> (connection ID out=w497:refnum<k5>, data out=w492:string, error out=w487:errorcluster)  [unwired: 2 in]
        n180 = Generate User Event(user event=w491, event data cluster=w492) -> (error out=w485:errorcluster)  [unwired: 2 in, 1 out]
        n181 = Equal?(x=w492, y="Stop") -> (x = y?=w500:bool)
        n182 = Merge Errors(w487, w484, w485) -> (w486:errorcluster)
        n183 = Or(x=w500, y=w499) -> (x .or. y?=w490:bool)
        n184 = case shown="False" w490 {
          tunnel: [w513 TCP_send_commands."Close TCP & Stop" ("Enum")] -> w489
          tunnel: w486 -> [w508 w525]
          tunnel: [w509 w524] -> w488
          tunnel: w483 -> [w511 _]
          tunnel: w482 -> [w507 _]
          frame False {
            n185 = Unbundle By Name(w508) -> ("code"=w510:i32)
            n186 = call "Ignore Specific Errors.vi"("error in (no error)"=w508, "Array"=i32[] [64, 66, 62, 1, 56]) -> ("error out"=w509:errorcluster)  [unwired: 8 in, 1 out]
            n187 = case shown="Default" w510 {
              tunnel: [TCP_send_commands."Init TCP" ("Enum") w518 TCP_send_commands."Init TCP" ("Enum")] -> w513
              tunnel: w511 -> [w516 _ w521]
              tunnel: w507 -> [_ w518 _]
              frame Default {
                n188 = property class="Enum (strict)"(reference=w516, "Value"=enum16{"Standalone", "UI Master", "UI Salve"}."Standalone" ("Value (Signaling)"), "Disabled"=u8 2) -> ()  [unwired: 1 in, 2 out]
              }
              frame 56 {
              }
              frame 1, 62, 64, 66 {
                n189 = property class="Enum (strict)"(reference=w521, "Value"=enum16{"Standalone", "UI Master", "UI Salve"}."Standalone" ("Value (Signaling)"), "Disabled"=u8 2) -> ()  [unwired: 1 in, 2 out]
              }
            }
          }
          frame True {
            n190 = call "Ignore Specific Errors.vi"("error in (no error)"=w525, "Array"=i32[] [64, 66, 62, 1, 56]) -> ("error out"=w524:errorcluster)  [unwired: 8 in, 1 out]
          }
        }
      }
      frame "Close TCP & Init" {
        n191 = TCP Close Connection(connection ID=w531) -> (connection ID out=w527:refnum<k5>, error out=w530:errorcluster)  [unwired: 2 in]
        n192 = call "Ignore Specific Errors.vi"("error in (no error)"=w530, "Array"=i32[] [1]) -> ("error out"=w529:errorcluster)  [unwired: 8 in, 1 out]
      }
    }
    n193 = call "error module.vi"("error in (no error)"=w434, "Enum"=error_module_commands."Process Errors") -> ("error out"=w436:errorcluster)  [unwired: 9 in]
  }
  n194 = Build Array(w9, w8, w7, w6) -> (w5:errorcluster[])
  n195 = Merge Errors(w5) -> (w4:errorcluster)
  n196 = call "error module.vi"("error in (no error)"=w4, "Enum"=error_module_commands."Cleanup References") -> ("error out"=w3:errorcluster)  [unwired: 9 in]
  n197 = call "error module.vi"("error in (no error)"=w3, "Enum"=error_module_commands."Report Errors") -> ()  [unwired: 9 in, 1 out]
